vi "MidBrain_checkoffMissions.vi"(10 "Mission QueueRef":T1, 11 "NotifierReff":T2) -> (2 "Waypoints Queue Out":refnum<queue>, 3 "BoatLocation Notifier Out":refnum<notifier>)   [LabVIEW 2013]
doc: "Removes waypoint from Queue if it's been checked off AND if there's still at least one element in the queue\n\n-Kaitlin (3/12/14)"
uses:
  Data/TypeDefs/Notifiers.ctl
  Data/TypeDefs/UTM Location.ctl
  Data/TypeDefs/Sail Set Suggestions.ctl
  Data/TypeDefs/Rudder Set Suggestions.ctl
  Data/TypeDefs/OverrideInformation.ctl
  Data/TypeDefs/OverrideMode.ctl
  Data/TypeDefs/MotorSetup.ctl
  Data/TypeDefs/DynamixelSetupInfo.ctl
  Data/TypeDefs/AirmarStatus.ctl
  Data/TypeDefs/HardwareOnline.ctl
  Data/TypeDefs/DynamixelCycleTracker.ctl
  Data/TypeDefs/RC Input Values.ctl
  Classes/Missions/GenericMission/GenericMission.lvclass
  Classes/Waypoint/Waypoint.lvclass
  Data/TypeDefs/Queues.ctl
  Classes/Obstacle/Obstacle.lvclass
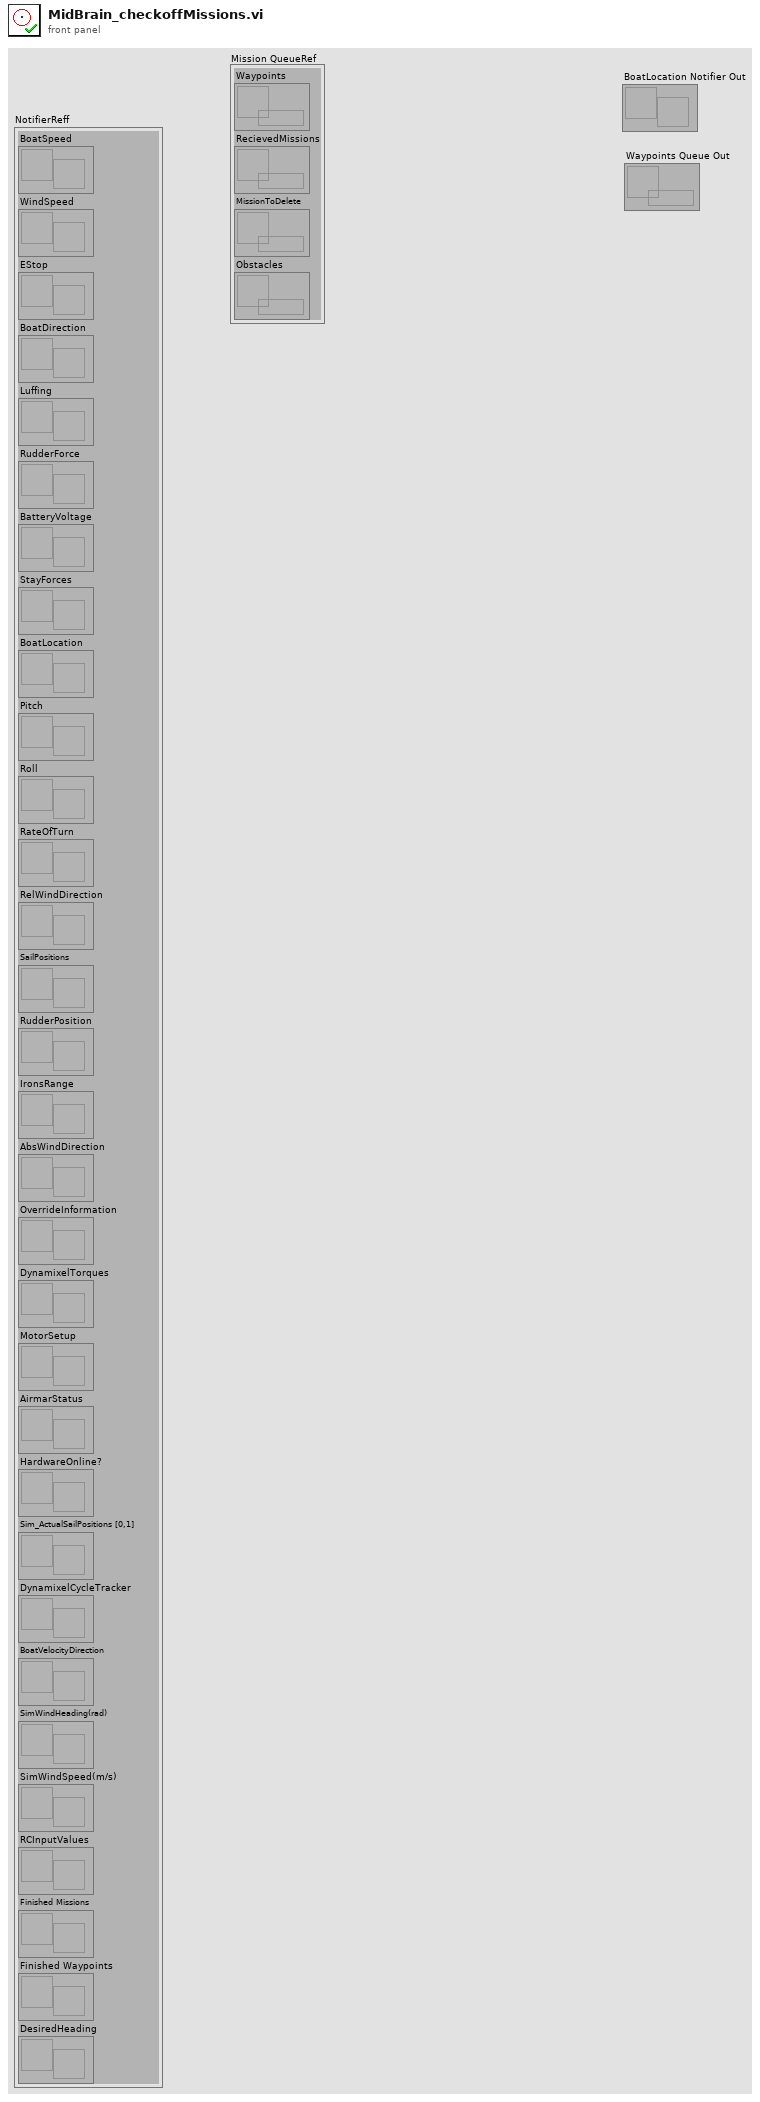
[diagram p1: front panel]
types:
  T1 = typedef "Queues.ctl" = cluster{"Waypoints":refnum<queue>, "RecievedMissions":refnum<queue>, "MissionToDelete":refnum<queue>, "Obstacles":refnum<queue>}
  T2 = typedef "Notifiers.ctl" = cluster{"BoatSpeed":refnum<notifier>, "WindSpeed":refnum<notifier>, "EStop":refnum<notifier>, "BoatDirection":refnum<notifier>, "Luffing":refnum<notifier>, "RudderForce":refnum<notifier>, "BatteryVoltage":refnum<notifier>, "StayForces":refnum<notifier>, "BoatLocation":refnum<notifier>, "Pitch":refnum<notifier>, "Roll":refnum<notifier>, "RateOfTurn":refnum<notifier>, "RelWindDirection":refnum<notifier>, "SailPositions":refnum<notifier>, "RudderPosition":refnum<notifier>, "IronsRange":refnum<notifier>, "AbsWindDirection":refnum<notifier>, "OverrideInformation":refnum<notifier>, "DynamixelTorques":refnum<notifier>, "MotorSetup":refnum<notifier>, "AirmarStatus":refnum<notifier>, "HardwareOnline?":refnum<notifier>, "Sim_ActualSailPositions [0,1]":refnum<notifier>, "DynamixelCycleTracker":refnum<notifier>, "BoatVelocityDirection":refnum<notifier>, "SimWindHeading(rad)":refnum<notifier>, "SimWindSpeed(m/s)":refnum<notifier>, "RCInputValues":refnum<notifier>, "Finished Missions":refnum<notifier>, "Finished Waypoints":refnum<notifier>, "DesiredHeading":refnum<notifier>}
  T3 = typedef "UTM Location.ctl" = cluster{"UTM Zone":dbl, "Hemisphere":enum16{"North", "South"}, "East":dbl, "North":dbl}
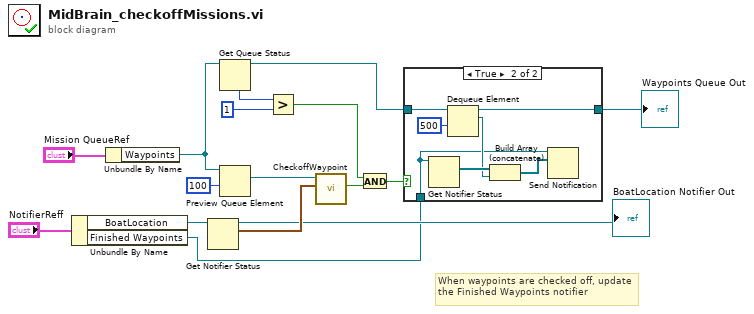
[diagram p0: block diagram]
diagram:
  # "When waypoints are checked off, update the Finished Waypoints notifier"
  n1 = Unbundle By Name("NotifierReff") -> ("BoatLocation"=w15:refnum<notifier>, "Finished Waypoints"=w1:refnum<notifier>)
  n2 = Unbundle By Name("Mission QueueRef") -> ("Waypoints"=w8:refnum<queue>)
  n3 = Get Notifier Status(notifier=w15) -> (notifier out=→"BoatLocation Notifier Out":refnum<notifier>, current notification=w12:T3)  [unwired: 1 in, 3 out]
  n4 = Get Queue Status(queue=w8) -> (queue out=w7:refnum<queue>, # elements in queue=w6:i32)  [unwired: 2 in, 6 out]
  n5 = Preview Queue Element(queue=w8, timeout in ms (-1)=100) -> (element=w11:refnum<class "Waypoint.lvclass">)  [unwired: 1 in, 3 out]
  n6 = Greater?(x=w6, y=1) -> (0:w3:bool)
  n7 = call "CheckoffWaypoint.vi"("CurrentLocation"=w12, "Waypoint In"=w11) -> ("Done?"=w4:bool)  [unwired: 7 in, 2 out]
  n8 = And(x=w3, y=w4) -> (x .and. y?=w2:bool)
  n9 = case shown="True" w2 {
    tunnel: w7 -> [w17 w24]
    tunnel: [w17 w23] -> w10
    tunnel: w1 -> [_ w18]
    frame False {
    }
    frame True {
      n10 = Get Notifier Status(notifier=w18) -> (current notification=w21:refnum<class "Waypoint.lvclass">[])  [unwired: 1 in, 4 out]
      n11 = Dequeue Element(queue=w24, timeout in ms (-1)=500) -> (queue out=w23:refnum<queue>, element=w20:refnum<class "Waypoint.lvclass">)  [unwired: 1 in, 2 out]
      n12 = Build Array (concatenate)(w21, w20) -> (w19:refnum<class "Waypoint.lvclass">[])
      n13 = Send Notification(notification=w19, notifier=w18) -> ()  [unwired: 1 in, 2 out]
    }
  }
  "Waypoints Queue Out" <- w10
